vi "OP400ZP_Plus1OuCrash.vi"(2 "IsStepOK?":bool, 3 "IN":T1=enum."Scan") -> (0 "OUT":T1=enum."Scan")   [LabVIEW 2020]
uses:
  OP400ZP_state.ctl
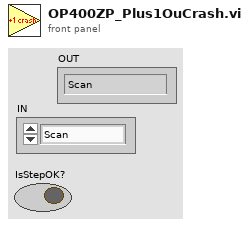
[diagram p1: front panel]
types:
  T1 = typedef "OP400ZP_state.ctl" = enum16{"Null", "Demarrage", "Init", "Scan", "Montage", "Conti", "Iso", "Vpack", "DataDyn", "Demontage", "Crash", "Next"}
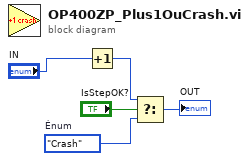
[diagram p0: block diagram]
diagram:
  w4 = OP400ZP_state."Crash"  # Énum
  n1 = Increment(x="IN") -> (x+1=w1:T1)
  n2 = Select(t=w1, s="IsStepOK?", f=w4) -> (s? t:f=→"OUT":T1)
